vi "Read CtlRef.vi"(8 "error in (no error)":errorcluster, 11 "ListboxEditCellMsg in":refnum<class "ListboxEditCellMsg.lvclass">) -> (0 "error out":errorcluster, 2 "CtlRef":refnum<vi>, 3 "ListboxEditCellMsg out":refnum<class "ListboxEditCellMsg.lvclass">)   [LabVIEW 2019, in "ActorEvents.lvlib" / "ListboxEditCellMsg.lvclass"]
uses:
  <vilib>/gpm_packages/@cs/mva-viewable/Source/ActorEvents/IEventAggregator Messages/ListboxEditCellMsg/ListboxEditCellMsg.lvclass
  <vilib>/gpm_packages/@cs/mva-viewable/Source/ActorEvents/IEventAggregator Messages/ListboxEditCellMsg/ListboxEditCellMsg.lvclass/ListboxEditCellMsg.ctl
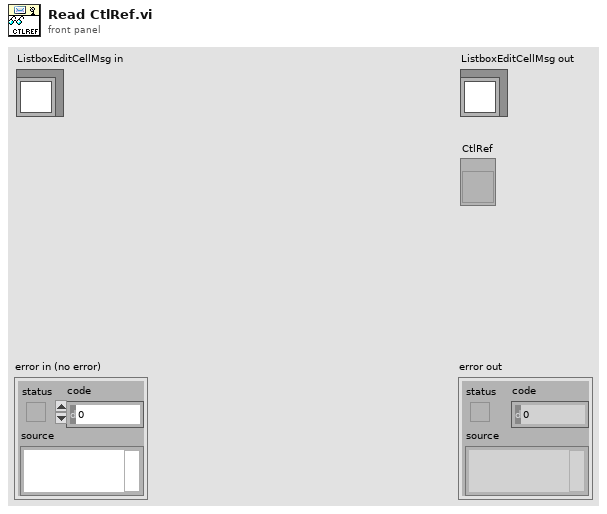
[diagram p1: front panel]
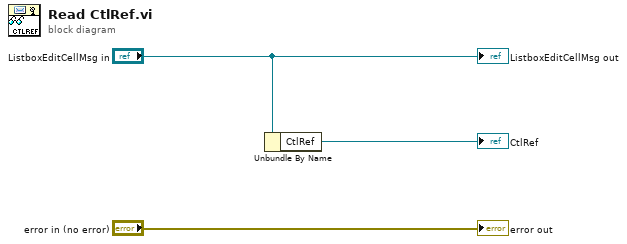
[diagram p0: block diagram]
diagram:
  n1 = Unbundle By Name("ListboxEditCellMsg in") -> ("CtlRef"=→"CtlRef":refnum<vi>)
  "error out" <- "error in (no error)"
  "ListboxEditCellMsg out" <- "ListboxEditCellMsg in"
